vi "yyllanalysis-CRC16_Calculator.vi"(5 "ByteOrder":bool, 6 "ReverseCRC":bool, 7 "LSB First":bool, 8 "Postcond":bool, 9 "Init":u16 format="%.0x", 10 "Polynom":u16=4129 format="%.0x", 11 "String in":string) -> (1 "Bytes":u8[](array[numeric]) format="%.0x", 2 "Numeric":u16 format="%.0x", 3 "CRC16 out":string)   [LabVIEW 2017]
doc: ">>>edit again by yyll---24.10\n\n\nThis is a general 16 bit CRC calculation VI.\n\nThe standard inputs will calculate the CRC with the following conditions:\n\nPolynom: x^16+x^12+x^5+1\nPrecondition: 0x0000\nPostcondition: not inverting\nMost significant bit of a byte first\nCRC output not bitwise reversed\nMost significant byte first\n\nThe input \"Check this message!\" will generate an output of 0x9E8F.\n\nThe VI was started by Shane aka shoneill in the NI Developer Zone. He implemented the HW like algorithm in the inner loop. Many thanks to him.\n\nThis VI was created and tested for the Intel plattform. I'm not sure that the byte order will be correct on a Motorola plattform."
panel:
  # "Input"
  # "Output"
  # "Conditioning"
  # "XorOut=FFFF?"
  # "https://www.sunshine2k.de/coding/javascript/crc/crc_js.html"
  # "Bitsequence"
  # "#YYLL Input reflected:"
  # "http://www.ip33.com/crc.html"
  # "#YYLL Result reflected:"
  # "https://www.crccalc.com/?crc=12423556ABCD4364FF&method=CRC-16/KERMIT&datatype=1&outtype=0"
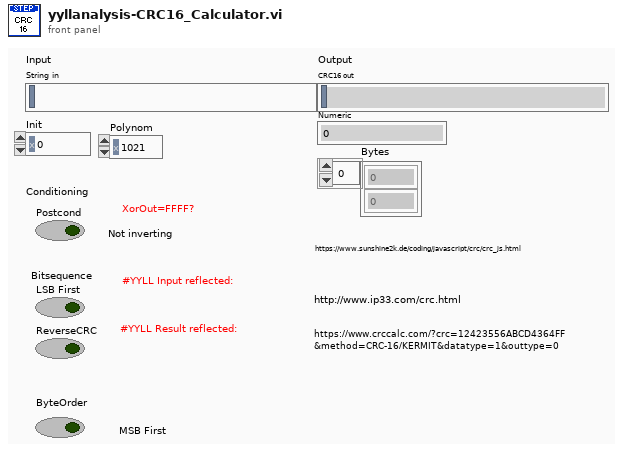
[diagram p1: front panel]
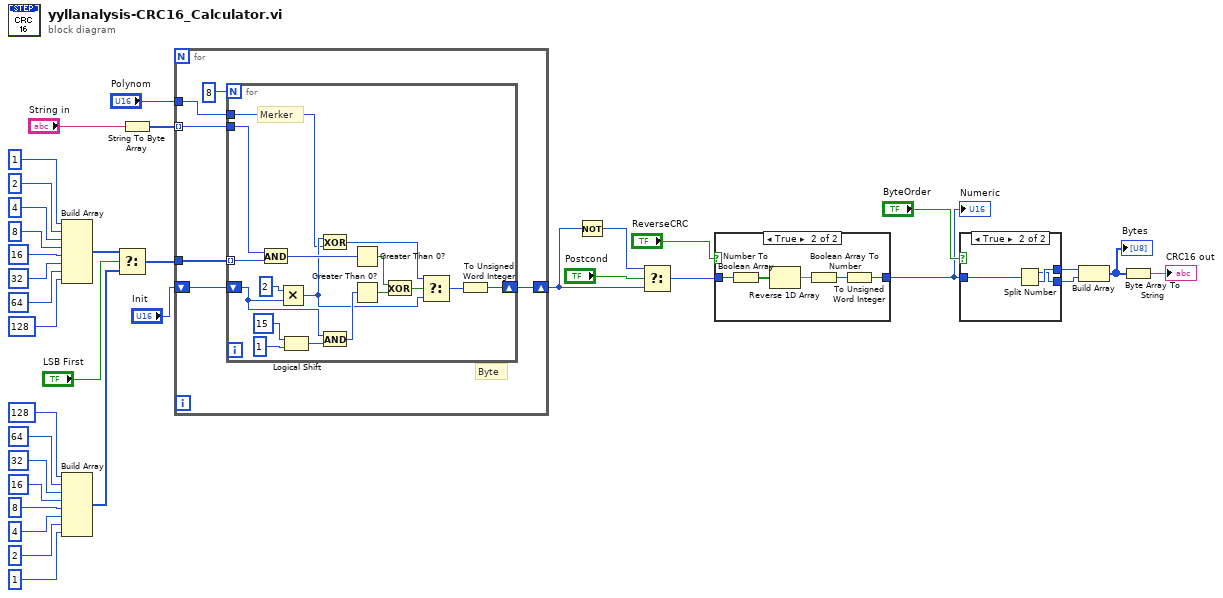
[diagram p0: block diagram]
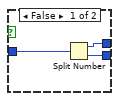
[diagram p2: hidden frame]
diagram:
  n1 = Build Array(u8 1, u8 2, u8 4, u8 8, u8 16, u8 32, u8 64, u8 128) -> (w13:u8[])
  n2 = Build Array(u8 128, u8 64, u8 32, u8 16, u8 8, u8 4, u8 2, u8 1) -> (w14:u8[])
  n3 = Select(t=w13, s="LSB First", f=w14) -> (s? t:f=w16:u8[])
  n4 = String To Byte Array(string="String in") -> (unsigned byte array=w34:u8[])
  n5 = for {
    shift-right: [w39] -> w12
    shift-left: "Init" -> [w41]
    tunnel: w34 -> [w38] mode=indexing
    tunnel: w16 -> [w37]
    tunnel: "Polynom" -> [w36]
    # "Byte"
    n6 = for {
      N: 8 -> [_]
      shift-right: [w57] -> w39
      shift-left: w41 -> [w47]
      tunnel: w37 -> [w48] mode=indexing
      tunnel: w38 -> [w43]
      tunnel: w36 -> [w42]
      # "Merker"
      n7 = And(x=w43, y=w48) -> (x .and. y?=w55:u8)
      n8 = Multiply(x=u16 2, y=w47) -> (x*y=w49:u16)
      n9 = Logical Shift(y=u16 15, x=u16 1) -> (x << y=w51:u16)
      n10 = Exclusive Or(1:w42, 2:w49) -> (0:w58:u16)
      n11 = And(x=w47, y=w51) -> (x .and. y?=w50:u16)
      n12 = Greater Than 0?(x=w55) -> (x > 0?=w54:bool)
      n13 = Greater Than 0?(x=w50) -> (x > 0?=w45:bool)
      n14 = Exclusive Or(1:w45, 2:w54) -> (0:w44:bool)
      n15 = Select(t=w58, s=w44, f=w49) -> (s? t:f=w56:u16)
      n16 = To Unsigned Word Integer(number=w56) -> (unsigned 16bit integer=w57:u16)
    }
  }
  n17 = Not(x=w12) -> (.not. x?=w11:u16)
  n18 = Select(t=w11, s="Postcond", f=w12) -> (s? t:f=w10:u16)
  n19 = case shown="True" "ReverseCRC" {
    tunnel: w10 -> [w59 w64]
    tunnel: [w59 w60] -> w2
    frame False {
    }
    frame True {
      n20 = Number To Boolean Array(number=w64) -> (Boolean array=w63:bool[])
      n21 = Reverse 1D Array(array=w63) -> (reversed array=w62:bool[])
      n22 = Boolean Array To Number(Boolean array=w62) -> (number=w61:u32)
      n23 = To Unsigned Word Integer(number=w61) -> (unsigned 16bit integer=w60:u16)
    }
  }
  "Numeric" <- w2
  n24 = case shown="True" "ByteOrder" {
    tunnel: w2 -> [w67 w70]
    tunnel: [w66 w69] -> w3
    tunnel: [w65 w68] -> w4
    frame False {
      n25 = Split Number(x=w67) -> (hi(x)=w66:u8, lo(x)=w65:u8)
    }
    frame True {
      n26 = Split Number(x=w70) -> (hi(x)=w68:u8, lo(x)=w69:u8)
    }
  }
  n27 = Build Array(w3, w4) -> (w6:u8[])
  "Bytes" <- w6
  n28 = Byte Array To String(unsigned byte array=w6) -> (string=→"CRC16 out":string)
